vi "Init.vi"(0 "input cluster":refnum<class "Application.lvclass">, 1 "This VI":refnum<vi>, 2 "Shield":refnum<vi>, 3 "SCORE":refnum<vi>, 5 "error in (no error)":errorcluster, 6 "STAR":refnum<vi>, 7 "Background":refnum<vi>, 8 "Score":refnum<vi>, 9 "Grapes":refnum<vi>, 10 "Board Game":refnum<vi>, 11 "Image Ring":refnum<vi>) -> (14 "Application out":refnum<class "Application.lvclass">, 19 "error out":errorcluster)   [LabVIEW 2021, in "Application.lvclass"]
uses:
  Application.lvclass
  Backgroud_v2.ctl
  GameEl_class/private/Enum Direction.ctl
  Snake_class/Snake.lvclass
  Fruit_class/Fruit.lvclass
  Shield/Shield.lvclass
  Grape/Grape.lvclass
  LVApp/Modules/Sound Manager/Typedefs/Sound Effects.ctl
  Mouse/Mouse.lvclass
  Cricket/Cricket.lvclass
  Star/Star.lvclass
  Application.lvclass/Application.ctl
  Star/Star.lvclass/Star.ctl
  Bomb/Bomb.lvclass
  Grape/Grape.lvclass/Grape.ctl
  Board Game_class/Board Game.lvclass/Board Game.ctl
  <vilib>/numeric/Random Number (Range) DBL.vi
  Board Game_class/Board Game.lvclass
  GameEl_class/GameEl.lvclass
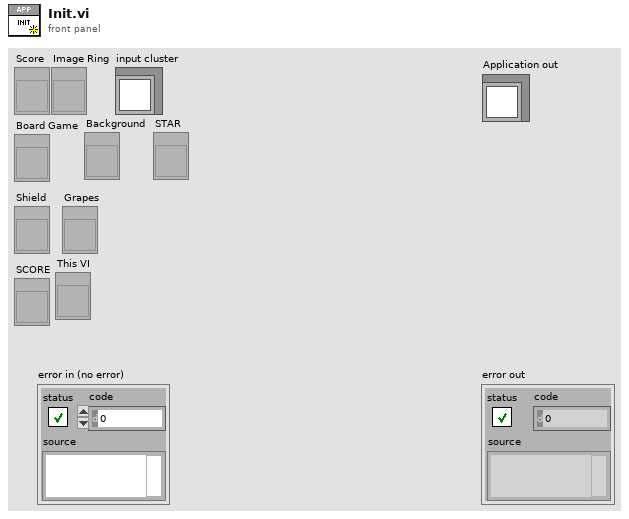
[diagram p1: front panel]
types:
  T1 = typedef "Sound Effects.ctl" = enum16{"Bomb In", "Bomb Out", "Bomb Touched", "Game Over", "Victory", "Eat", "10 Fruits", "Eat2", "Eat3", "Eat4", "MaxShield", "Shield", "10p", "Grape In", "Grape Out", "20p", "30p", "40p", "50p", "60p", "70p", "80p", "90p", "100p", "All shields cracked", "Mouse In", "Mouse Out", "Mouse Eaten", "Grape Eaten", "States Recover", "Broken Shield", "Bonus", "Happy Time", "explode", "Game over musica", "Back Music", "Shield Catch", "Evil lough", "Cricket In", "Cricket eaten", "Lets Go", "Jump1", "Jump2", "Jump3", "Unstoppable", "Troll Music", "winner"}
  T2 = typedef "GameEl.lvclass/Enum Direction.ctl" = enum16{"Up", "Down", "Forward", "Backward"}
  T3 = cluster{"millisecond timer value":u32, "Elapsed":u32}
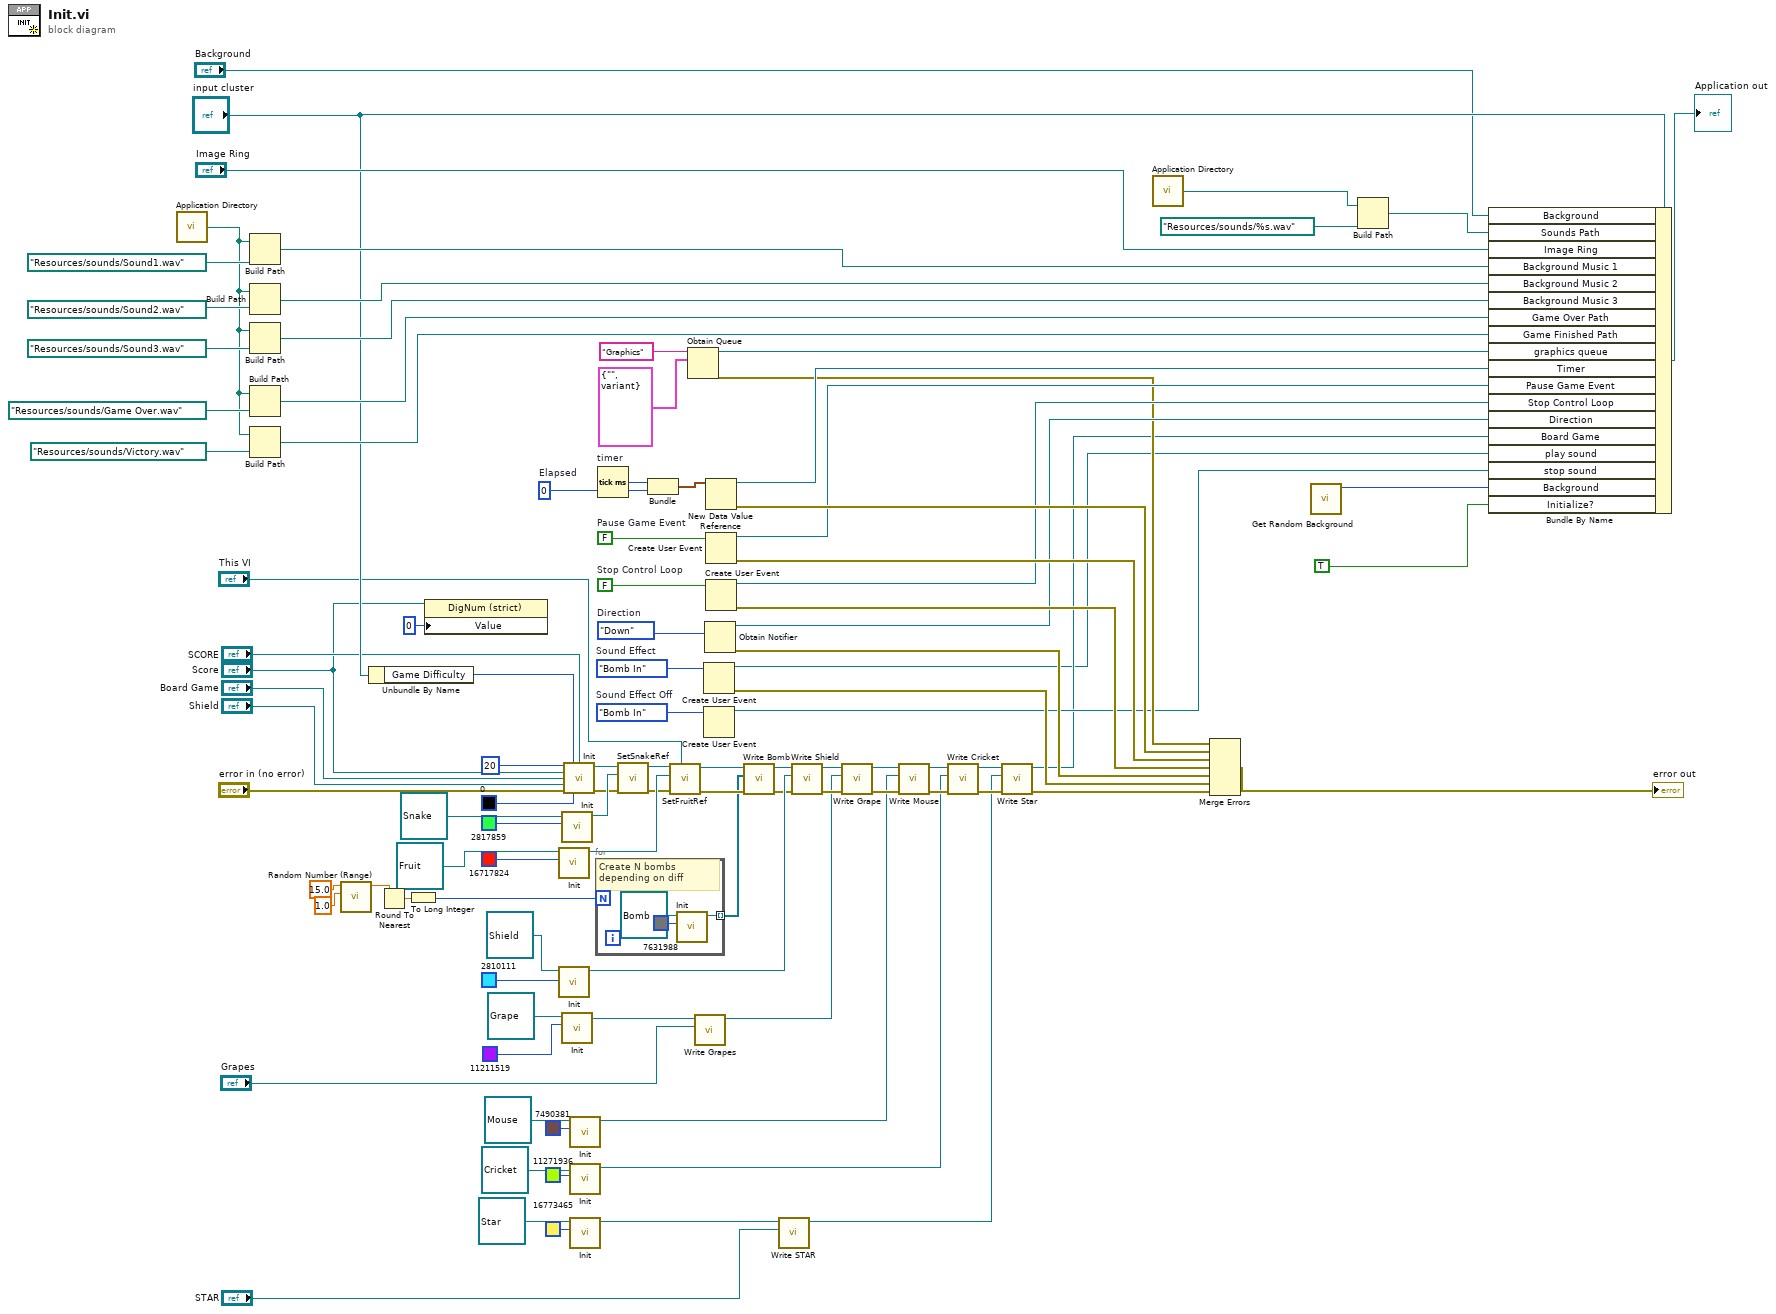
[diagram p0: block diagram]
diagram:
  w21 = u32 0  # Elapsed
  w32 = Sound_Effects."Bomb In"  # Sound Effect Off
  w43 = Sound_Effects."Bomb In"  # Sound Effect
  w91 = FALSE  # Pause Game Event
  w92 = FALSE  # Stop Control Loop
  w99 = Enum_Direction."Down"  # Direction
  n1 = call <vilib>:"Application Directory.vi"() -> ("Application Directory"=w57:path)
  n2 = Build Path(base path=w57, name or relative path=path "Resources/sounds/Sound1.wav") -> (appended path=w78:path)
  n3 = Build Path(base path=w57, name or relative path=path "Resources/sounds/Sound2.wav") -> (appended path=w77:path)
  n4 = Build Path(base path=w57, name or relative path=path "Resources/sounds/Sound3.wav") -> (appended path=w75:path)
  n5 = Build Path(base path=w57, name or relative path=path "Resources/sounds/Game Over.wav") -> (appended path=w81:path)
  n6 = Build Path(base path=w57, name or relative path=path "Resources/sounds/Victory.wav") -> (appended path=w80:path)
  n7 = call-poly <vilib>:"Random Number (Range).vi"("lower bound (0)"=1.0 ("Low"), "upper bound (100)"=15.0 ("High")) -> ("number"=w27:dbl)  [unwired: 9 in]
  n8 = Unbundle By Name("input cluster") -> ("Game Difficulty"=w69:u32)
  n9 = Round To Nearest(number=w27) -> (nearest integer value=w26:dbl)
  n10 = To Long Integer(number=w26) -> (32bit integer=w23:i32)
  n11 = property class="DigNum (strict)"(reference="Score", "Value"=u16 0) -> ()  [unwired: 1 in, 2 out]
  n12 = call-dynamic "Init.vi"("Colour"=u32 16717824, "GameEl in"=refnum<class "Fruit.lvclass"> refnum ("Object in")) -> ("GameEl out"=w98:refnum<class "Fruit.lvclass">)  [unwired: 8 in, 1 out]
  n13 = call-dynamic "Init.vi"("Colour"=u32 2810111, "GameEl in"=refnum<class "Shield.lvclass"> refnum ("Shield in")) -> ("GameEl out"=w61:refnum<class "Shield.lvclass">)  [unwired: 8 in, 1 out]
  n14 = call-dynamic "Init.vi"("Colour"=u32 2817859, "Snake In"=refnum<class "Snake.lvclass"> refnum) -> ("object out"=w100:refnum<class "Snake.lvclass">)  [unwired: 8 in, 1 out]
  n15 = call-dynamic "Init.vi"("Colour"=u32 11211519, "GameEl in"=refnum<class "Grape.lvclass"> refnum ("Grape.lvclass")) -> ("GameEl out"=w46:refnum<class "Grape.lvclass">)  [unwired: 8 in, 1 out]
  n16 = call "Init.vi"("Size"=u16 20, "Game Difficulty Out"=w69, "SCORE"="SCORE", "Score"="Score", "Board Game"="Board Game", "Shield"="Shield", "error in (no error)"="error in (no error)", "Colour"=u32 0) -> ("Board Game out"=w93:refnum<class "Board Game.lvclass">, "error out"=w97:errorcluster)  [unwired: 6 in]
  n17 = call-dynamic "Init.vi"("Colour"=u32 7490381, "GameEl in"=refnum<class "Mouse.lvclass"> refnum ("Mouse.lvclass")) -> ("GameEl out"=w34:refnum<class "Mouse.lvclass">)  [unwired: 8 in, 1 out]
  n18 = call-dynamic "Init.vi"("Colour"=u32 11271936, "GameEl in"=refnum<class "Cricket.lvclass"> refnum ("Cricket.lvclass")) -> ("GameEl out"=w16:refnum<class "Cricket.lvclass">)  [unwired: 8 in, 1 out]
  n19 = call-dynamic "Init.vi"("Colour"=u32 16773465, "GameEl in"=refnum<class "Star.lvclass"> refnum ("Star.lvclass")) -> ("GameEl out"=w7:refnum<class "Star.lvclass">)  [unwired: 8 in, 1 out]
  n20 = for {
    N: w23 -> [_]
    tunnel: [w106] -> w68 mode=indexing
    # "Create N bombs\ndepending on diff"
    n21 = call-dynamic "Init.vi"("Colour"=u32 7631988, "GameEl in"=refnum<class "Bomb.lvclass"> refnum ("Bomb In")) -> ("GameEl out"=w106:refnum<class "Bomb.lvclass">)  [unwired: 8 in, 1 out]
  }
  n22 = Tick Count (ms) "timer"() -> (millisecond timer value=w85:u32)
  n23 = call-dynamic "SetSnakeRef.vi"("Error In"=w97, "SnakeRef"=w100, "object in"=w93) -> ("Error Out"=w95:errorcluster, "object out"=w94:refnum<class "Board Game.lvclass">)  [unwired: 7 in]
  n24 = Bundle("millisecond timer value"=w85, "Elapsed"=w21) -> (w22:T3)  [unwired: 1 in]
  n25 = call-dynamic "SetFruitRef.vi"("This VI"="This VI", "Error In"=w95, "FruitRef"=w98, "object in"=w94) -> ("Error Out"=w73:errorcluster, "object out"=w74:refnum<class "Board Game.lvclass">)  [unwired: 6 in]
  n26 = Obtain Queue(name (unnamed)="Graphics", element data type=cluster{"Message":string, "Data":variant} {"Message"="", "Data"=variant}) -> (queue out=w66:refnum<queue>, error out=w38:errorcluster)  [unwired: 3 in, 1 out]
  n27 = call "Write Grapes.vi"("Grapes"="Grapes", "Grape in"=w46) -> ("Grape out"=w45:refnum<class "Grape.lvclass">)  [unwired: 8 in, 1 out]
  n28 = Create User Event(user event datatype=w43) -> (user event=w6:refnum<user-event>, error out=w39:errorcluster)  [unwired: 1 in]
  n29 = Create User Event(user event datatype=w32) -> (user event=w31:refnum<user-event>)  [unwired: 1 in, 1 out]
  n30 = Obtain Notifier(notification data type=w99) -> (notifier out=w62:refnum<notifier>, error out=w88:errorcluster)  [unwired: 3 in, 1 out]
  n31 = New Data Value Reference(data value=w22) -> (data value reference=w65:refnum<data-value>, error out=w86:errorcluster)  [unwired: 1 in]
  n32 = Create User Event(user event datatype=w91) -> (user event=w64:refnum<user-event>, error out=w90:errorcluster)  [unwired: 1 in]
  n33 = Create User Event(user event datatype=w92) -> (user event=w63:refnum<user-event>, error out=w89:errorcluster)  [unwired: 1 in]
  n34 = call "Write Bomb.vi"("error in (no error)"=w73, "Array"=w68, "Board Game in"=w74) -> ("error out"=w58:errorcluster, "Board Game out"=w60:refnum<class "Board Game.lvclass">)  [unwired: 7 in]
  n35 = call "Write STAR.vi"("STAR"="STAR", "Star in"=w7) -> ("Star out"=w4:refnum<class "Star.lvclass">)  [unwired: 8 in, 1 out]
  n36 = call "Write Shield.vi"("error in (no error)"=w58, "Shield.lvclass"=w61, "Board Game in"=w60) -> ("error out"=w47:errorcluster, "Board Game out"=w59:refnum<class "Board Game.lvclass">)  [unwired: 7 in]
  n37 = call "Write Grape.vi"("error in (no error)"=w47, "Grape.lvclass"=w45, "Board Game in"=w59) -> ("error out"=w37:errorcluster, "Board Game out"=w48:refnum<class "Board Game.lvclass">)  [unwired: 7 in]
  n38 = call "Write Mouse.vi"("error in (no error)"=w37, "Mouse.lvclass"=w34, "Board Game in"=w48) -> ("error out"=w36:errorcluster, "Board Game out"=w17:refnum<class "Board Game.lvclass">)  [unwired: 7 in]
  n39 = call "Write Cricket.vi"("error in (no error)"=w36, "Cricket.lvclass"=w16, "Board Game in"=w17) -> ("error out"=w18:errorcluster, "Board Game out"=w9:refnum<class "Board Game.lvclass">)  [unwired: 7 in]
  n40 = call "Write Star.vi"("error in (no error)"=w18, "Star.lvclass"=w4, "Board Game in"=w9) -> ("error out"=w10:errorcluster, "Board Game out"=w8:refnum<class "Board Game.lvclass">)  [unwired: 7 in]
  n41 = call <vilib>:"Application Directory.vi"() -> ("Application Directory"=w42:path)
  n42 = Merge Errors(w38, w86, w90, w89, w88, w39, w10) -> (→"error out":errorcluster)
  n43 = call "Get Random Background.vi"() -> ("Numeric"=w24:u16)  [unwired: 11 in]
  n44 = Build Path(base path=w42, name or relative path=path "Resources/sounds/%s.wav") -> (appended path=w40:path)
  n45 = Bundle By Name(cluster="input cluster", "Background"="Background", "Sounds Path"=w40, "Image Ring"="Image Ring", "Background Music 1"=w78, "Background Music 2"=w77, "Background Music 3"=w75, "Game Over Path"=w81, "Game Finished Path"=w80, "graphics queue"=w66, "Timer"=w65, "Pause Game Event"=w64, "Stop Control Loop"=w63, "Direction"=w62, "Board Game"=w8, "play sound"=w6, "stop sound"=w31, "Background"=w24, "Initialize?"=TRUE) -> (→"Application out":refnum<class "Application.lvclass">)
